vi "ToString.vi"(8 "error in (no error)":errorcluster, 11 "Error in":refnum<class "Error.lvclass">) -> (0 "error out":errorcluster, 2 "String":string, 3 "Error out":refnum<class "Error.lvclass">)   [LabVIEW 2017, in "Transparent Assertions.lvlib" / "Error.lvclass"]
doc: "Returns a string representation of the object."
uses:
  Error.lvclass
  Error.lvclass/Error.ctl
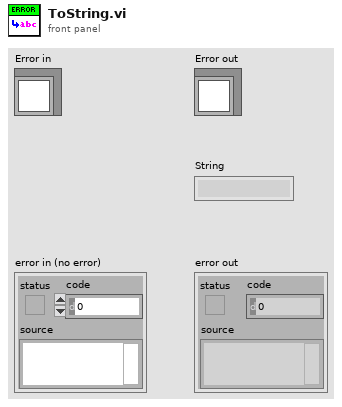
[diagram p1: front panel]
types:
  T1 = typedef "Transparent Assertions.lvlib/Error.lvclass/ErrorType.ctl" = enum16{"error", "warning", "no error"}
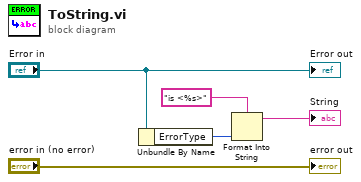
[diagram p0: block diagram]
diagram:
  n1 = Unbundle By Name("Error in") -> ("ErrorType"=w3:T1)
  n2 = Format Into String(format string="is <%s>" ("String"), w3) -> (resulting string=→"String":string)  [unwired: 2 in, 1 out]
  "error out" <- "error in (no error)"
  "Error out" <- "Error in"
